vi "cmd获取空闲端口.vi"(10 "地址":enum16{"当前IP", "localhost"}(ring), 11 "协议":enum16{"TCP", "UDP"}(ring)) -> (2 "空闲端口":i32, 3 "占用的端口":u16[](array[numeric]), 4 "网络连接可用?":bool)   [LabVIEW 2017]
panel:
  out "占用数量":i32
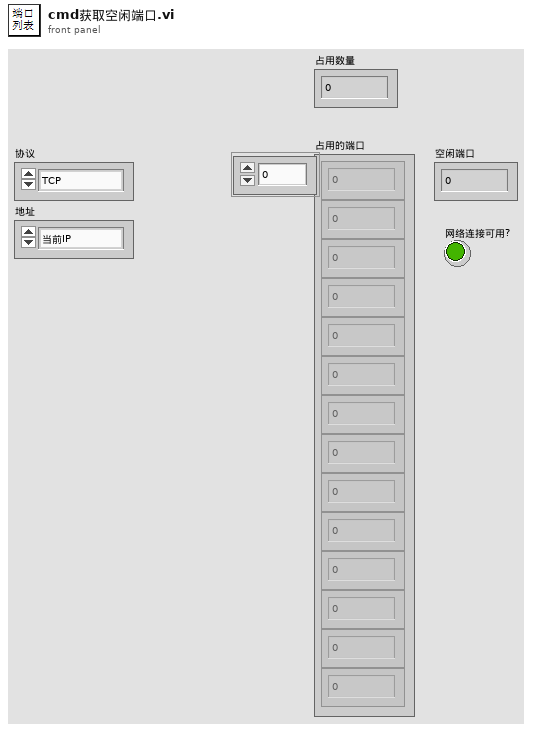
[diagram p1: front panel]
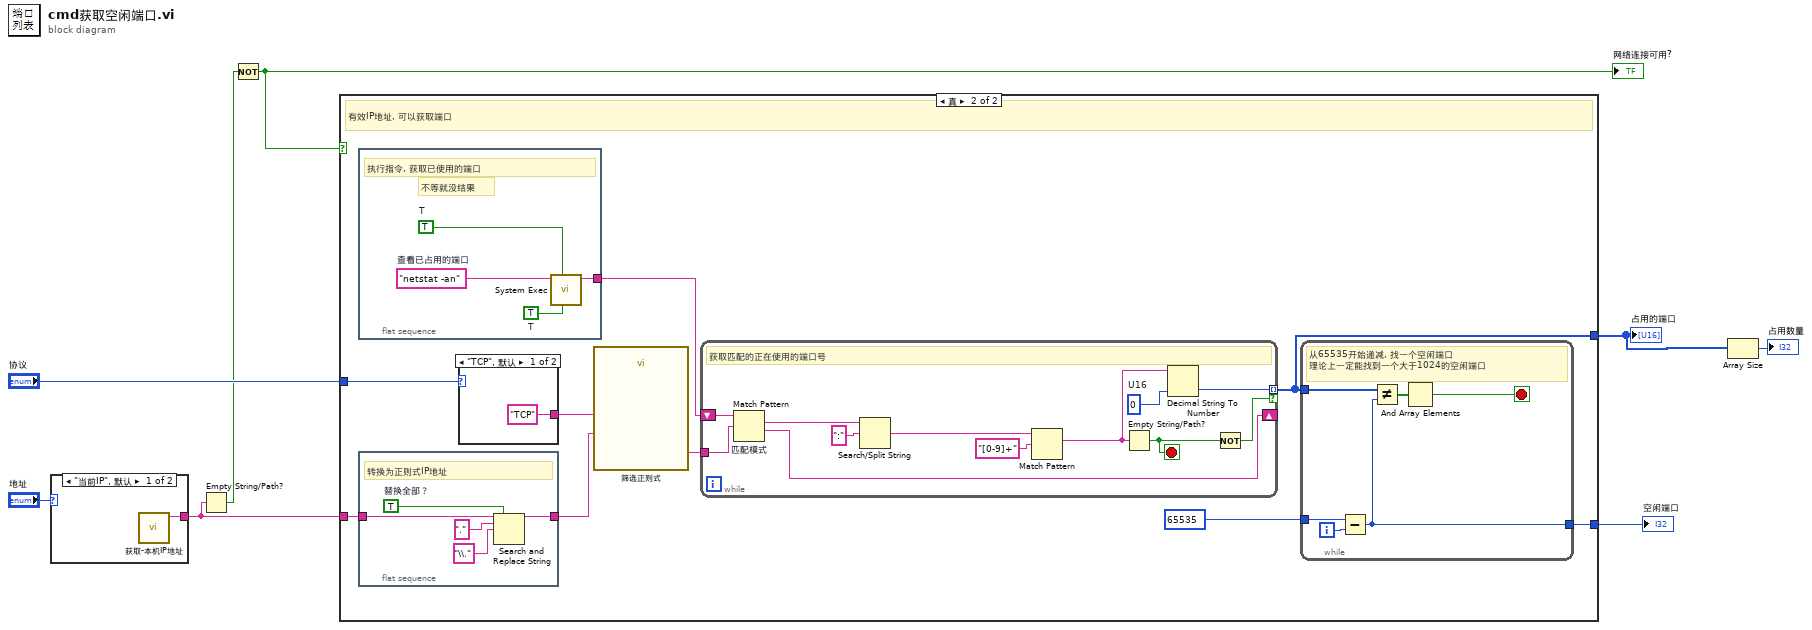
[diagram p0: block diagram]
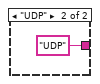
[diagram p3: hidden frame]
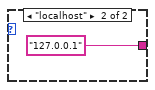
[diagram p4: hidden frame]
diagram:
  n1 = case shown="\"当前IP\", 默认" "地址" {
    tunnel: [w9 "127.0.0.1" ("正则表达式")] -> w6
    frame "当前IP", Default {
      n2 = call "获取-本机IP地址.vi"() -> ("本机IP"=w9:string)  [unwired: 10 in, 1 out]
    }
    frame "localhost" {
    }
  }
  n3 = Empty String/Path?(string/path=w6) -> (empty?=w5:bool)
  n4 = Not(x=w5) -> (.not. x?=w4:bool)
  "网络连接可用?" <- w4
  n5 = case shown="真" w4 {
    tunnel: "协议" -> [_ w19]
    tunnel: [_ w13] -> w2
    tunnel: w6 -> [_ w14]
    tunnel: [_ w12] -> w3
    frame False {
      # "无效IP地址, 说明现在没有连接任何网络, 不执行"
    }
    frame True {
      # "有效IP地址, 可以获取端口"
      n6 = flat-sequence {
        tunnel: [w26] -> w15
        frame #0 {
          w27 = TRUE  # T
          w28 = TRUE  # T
          w29 = "netstat -an"  # 查看已占用的端口
          # "不等就没结果"
          # "执行指令, 获取已使用的端口"
          n7 = call <vilib>:"System Exec.vi"("run minimized? (F)"=w28, "wait until completion? (T)"=w27, "command line"=w29) -> ("standard output"=w26:string)  [unwired: 5 in, 3 out]
        }
      }
      n8 = flat-sequence {
        tunnel: [w45] -> w17
        tunnel: w14 -> [w44]
        frame #0 {
          w48 = TRUE  # 替换全部？
          # "转换为正则式IP地址"
          n9 = Search and Replace String(replace all?=w48, input string=w44, search string="." ("搜索字符串"), replace string="\\." ("替换字符串(\"\")")) -> (result string=w45:string)  [unwired: 4 in, 3 out]
        }
      }
      n10 = case shown="\"TCP\", 默认" w19 {
        tunnel: ["TCP" ("正则表达式") "UDP" ("正则表达式")] -> w18
        frame "TCP", Default {
        }
        frame "UDP" {
        }
      }
      n11 = call "筛选正则式"("协议"=w18, "正则IP地址"=w17) -> ("Result"=w16:string)  [unwired: 12 in, 1 out]
      n12 = while {
        tunnel: w16 -> [w41]
        shift-right: [w39] -> _
        shift-left: w15 -> [w40]
        tunnel: [w33] -> w13 mode=indexing if=w31
        stop <- w30 stop-if-true
        w34 = u16 0  # U16
        # "获取匹配的正在使用的端口号"
        n13 = Match Pattern "匹配模式"(string=w40, regular expression=w41) -> (match substring=w37:string, after substring=w39:string)  [unwired: 1 in, 2 out]
        n14 = Search/Split String(string=w37, search string/char (-)=":" ("搜索字符串/字符(-)")) -> (match + rest of string=w35:string)  [unwired: 1 in, 2 out]
        n15 = Match Pattern(string=w35, regular expression="[0-9]+" ("正则表达式")) -> (match substring=w32:string)  [unwired: 1 in, 3 out]
        n16 = Empty String/Path?(string/path=w32) -> (empty?=w30:bool)
        n17 = Decimal String To Number(string=w32, default (0L)=w34) -> (number=w33:u16)  [unwired: 1 in, 1 out]
        n18 = Not(x=w30) -> (.not. x?=w31:bool)
      }
      n19 = while {
        tunnel: u16 65535 -> [w24]
        tunnel: w13 -> [w23]
        tunnel: [w20] -> w12
        i -> [w25]
        stop <- w21 stop-if-true
        # "从65535开始递减, 找一个空闲端口\n理论上一定能找到一个大于1024的空闲端口"
        n20 = Subtract(x=w24, y=w25) -> (x-y=w20:i32)
        n21 = Not Equal?(x=w23, y=w20) -> (x != y?=w22:bool[])
        n22 = And Array Elements(Boolean array=w22) -> (logical AND=w21:bool)
      }
    }
  }
  "占用的端口" <- w2
  "空闲端口" <- w3
  n23 = Array Size(array=w2) -> (size(s)=→"占用数量":i32)
